vi "IsCurrStepLessThenSize.vi"(11 "Curr step":i32) -> (3 "Boolean":bool)   [LabVIEW 2017]
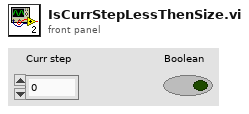
[diagram p1: front panel]
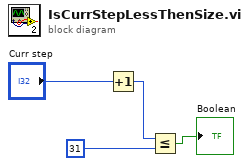
[diagram p0: block diagram]
diagram:
  n1 = Increment(x="Curr step") -> (x+1=w2:i32)
  n2 = Less Or Equal?(x=w2, y=31) -> (x <= y?=→"Boolean":bool)
